vi "S2C_FPGA_WritePort.vi"(8 "Data":u8, 10 "Port":T1(ring), 11 "Connector":enum8{"Conn_0", "Conn_1", "Conn_2"}(ring)) -> ()   [LabVIEW 2015]
uses:
  <vilib>/eio/EIONode/EIONode.xnode
  <vilib>/rvi/eio/common/nirviEmuTemplateMethod_errors.vi
  S2C_FPGA_Global.vi
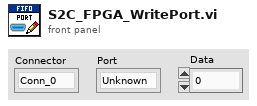
[diagram p1: front panel]
types:
  T1 = enum8{"Unknown", "Port_0", "Port_1", "Port_2", "Port_3", "Port_4"}
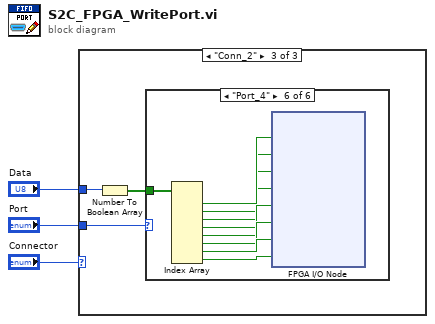
[diagram p0: block diagram]
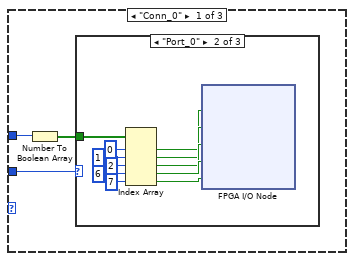
[diagram p2: hidden frame]
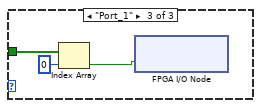
[diagram p4: hidden frame]
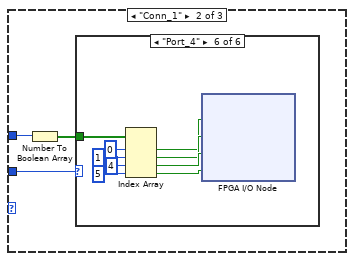
[diagram p5: hidden frame]
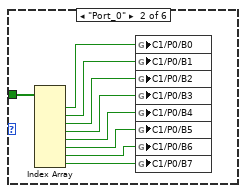
[diagram p7: hidden frame]
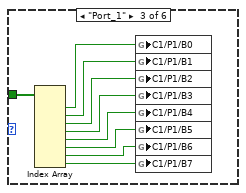
[diagram p8: hidden frame]
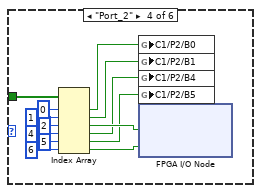
[diagram p9: hidden frame]
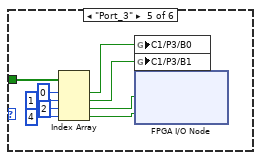
[diagram p10: hidden frame]
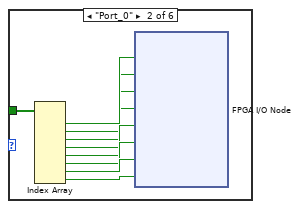
[diagram p12: hidden frame]
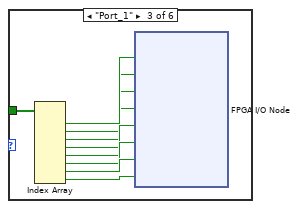
[diagram p13: hidden frame]
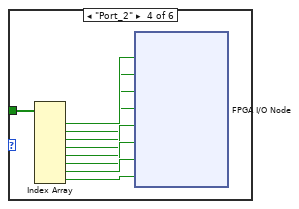
[diagram p14: hidden frame]
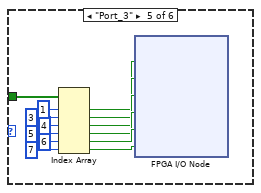
[diagram p15: hidden frame]
diagram:
  n1 = case shown="\"Conn_2\"" "Connector" {
    tunnel: "Data" -> [w6 w23 w75]
    tunnel: "Port" -> [w4 w21 w73]
    frame "Conn_0" {
      n2 = Number To Boolean Array(number=w6) -> (Boolean array=w5:bool[])
      n3 = case shown="\"Port_0\"" w4 {
        tunnel: w5 -> [_ w17 w20]
        frame "Unknown", Default {
        }
        frame "Port_0" {
          n4 = Index Array(array=w17, index #1=0 ("index"), index #2=1 ("index"), index #3=2 ("index"), index #4=6 ("index"), index #5=7 ("index")) -> (element #1=w7:bool, element #2=w8:bool, element #3=w9:bool, element #4=w10:bool, element #5=w11:bool)
          n5 = xnode "FPGA I/O Node"("C0/P0/B0"=w7, "C0/P0/B1"=w8, "C0/P0/B2"=w9, "C0/P0/B6"=w10, "C0/P0/B7"=w11) -> ()  [unwired: 5 in, 5 out]
        }
        frame "Port_1" {
          n6 = Index Array(array=w20, index=0) -> (element=w18:bool)
          n7 = xnode "FPGA I/O Node"("C0/P1/B0"=w18) -> ()  [unwired: 1 in, 1 out]
        }
      }
    }
    frame "Conn_1" {
      n8 = Number To Boolean Array(number=w23) -> (Boolean array=w22:bool[])
      n9 = case shown="\"Port_4\"" w21 {
        tunnel: w22 -> [_ w32 w41 w49 w59 w68]
        frame "Unknown", Default {
        }
        frame "Port_0" {
          n10 = Index Array(array=w32) -> (element #1=w30:bool, element #2=w29:bool, element #3=w28:bool, element #4=w27:bool, element #5=w26:bool, element #6=w25:bool, element #7=w24:bool, element #8=w31:bool)  [unwired: 8 in]
          n11 = global write "S2C_FPGA_Global.vi" "C1/P0/B0"(w30) -> ()
          n12 = global write "S2C_FPGA_Global.vi" "C1/P0/B1"(w29) -> ()
          n13 = global write "S2C_FPGA_Global.vi" "C1/P0/B2"(w28) -> ()
          n14 = global write "S2C_FPGA_Global.vi" "C1/P0/B3"(w27) -> ()
          n15 = global write "S2C_FPGA_Global.vi" "C1/P0/B4"(w26) -> ()
          n16 = global write "S2C_FPGA_Global.vi" "C1/P0/B5"(w25) -> ()
          n17 = global write "S2C_FPGA_Global.vi" "C1/P0/B6"(w24) -> ()
          n18 = global write "S2C_FPGA_Global.vi" "C1/P0/B7"(w31) -> ()
        }
        frame "Port_1" {
          n19 = Index Array(array=w41) -> (element #1=w39:bool, element #2=w38:bool, element #3=w37:bool, element #4=w36:bool, element #5=w35:bool, element #6=w34:bool, element #7=w33:bool, element #8=w40:bool)  [unwired: 8 in]
          n20 = global write "S2C_FPGA_Global.vi" "C1/P1/B0"(w39) -> ()
          n21 = global write "S2C_FPGA_Global.vi" "C1/P1/B1"(w38) -> ()
          n22 = global write "S2C_FPGA_Global.vi" "C1/P1/B2"(w37) -> ()
          n23 = global write "S2C_FPGA_Global.vi" "C1/P1/B3"(w36) -> ()
          n24 = global write "S2C_FPGA_Global.vi" "C1/P1/B4"(w35) -> ()
          n25 = global write "S2C_FPGA_Global.vi" "C1/P1/B5"(w34) -> ()
          n26 = global write "S2C_FPGA_Global.vi" "C1/P1/B6"(w33) -> ()
          n27 = global write "S2C_FPGA_Global.vi" "C1/P1/B7"(w40) -> ()
        }
        frame "Port_2" {
          n28 = Index Array(array=w49, index #1=0 ("index"), index #2=1 ("index"), index #3=2 ("index"), index #4=4 ("index"), index #5=5 ("index"), index #6=6 ("index")) -> (element #1=w48:bool, element #2=w47:bool, element #3=w46:bool, element #4=w44:bool, element #5=w43:bool, element #6=w42:bool)
          n29 = global write "S2C_FPGA_Global.vi" "C1/P2/B0"(w48) -> ()
          n30 = global write "S2C_FPGA_Global.vi" "C1/P2/B1"(w47) -> ()
          n31 = global write "S2C_FPGA_Global.vi" "C1/P2/B4"(w44) -> ()
          n32 = global write "S2C_FPGA_Global.vi" "C1/P2/B5"(w43) -> ()
          n33 = xnode "FPGA I/O Node"("C1/P2/B2"=w46, "C1/P2/B6"=w42) -> ()  [unwired: 2 in, 2 out]
        }
        frame "Port_3" {
          n34 = Index Array(array=w59, index #1=0 ("index"), index #2=1 ("index"), index #3=2 ("index"), index #4=4 ("index")) -> (element #1=w58:bool, element #2=w57:bool, element #3=w56:bool, element #4=w55:bool)
          n35 = global write "S2C_FPGA_Global.vi" "C1/P3/B0"(w58) -> ()
          n36 = global write "S2C_FPGA_Global.vi" "C1/P3/B1"(w57) -> ()
          n37 = xnode "FPGA I/O Node"("C1/P3/B2"=w56, "C1/P3/B4"=w55) -> ()  [unwired: 2 in, 2 out]
        }
        frame "Port_4" {
          n38 = Index Array(array=w68, index #1=0 ("index"), index #2=1 ("index"), index #3=4 ("index"), index #4=5 ("index")) -> (element #1=w64:bool, element #2=w65:bool, element #3=w66:bool, element #4=w67:bool)
          n39 = xnode "FPGA I/O Node"("C1/P4/B0"=w64, "C1/P4/B1"=w65, "C1/P4/B4"=w66, "C1/P4/B5"=w67) -> ()  [unwired: 4 in, 4 out]
        }
      }
    }
    frame "Conn_2" {
      n40 = Number To Boolean Array(number=w75) -> (Boolean array=w74:bool[])
      n41 = case shown="\"Port_4\"" w73 {
        tunnel: w74 -> [_ w84 w93 w102 w110 w124]
        frame "Unknown", Default {
        }
        frame "Port_0" {
          n42 = Index Array(array=w84) -> (element #1=w83:bool, element #2=w76:bool, element #3=w77:bool, element #4=w78:bool, element #5=w79:bool, element #6=w80:bool, element #7=w81:bool, element #8=w82:bool)  [unwired: 8 in]
          n43 = xnode "FPGA I/O Node"("C2/P0/B0"=w83, "C2/P0/B1"=w76, "C2/P0/B2"=w77, "C2/P0/B3"=w78, "C2/P0/B4"=w79, "C2/P0/B5"=w80, "C2/P0/B6"=w81, "C2/P0/B7"=w82) -> ()  [unwired: 8 in, 8 out]
        }
        frame "Port_1" {
          n44 = Index Array(array=w93) -> (element #1=w92:bool, element #2=w85:bool, element #3=w86:bool, element #4=w87:bool, element #5=w88:bool, element #6=w89:bool, element #7=w90:bool, element #8=w91:bool)  [unwired: 8 in]
          n45 = xnode "FPGA I/O Node"("C2/P1/B0"=w92, "C2/P1/B1"=w85, "C2/P1/B2"=w86, "C2/P1/B3"=w87, "C2/P1/B4"=w88, "C2/P1/B5"=w89, "C2/P1/B6"=w90, "C2/P1/B7"=w91) -> ()  [unwired: 8 in, 8 out]
        }
        frame "Port_2" {
          n46 = Index Array(array=w102) -> (element #1=w101:bool, element #2=w94:bool, element #3=w95:bool, element #4=w96:bool, element #5=w97:bool, element #6=w98:bool, element #7=w99:bool, element #8=w100:bool)  [unwired: 8 in]
          n47 = xnode "FPGA I/O Node"("C2/P2/B0"=w101, "C2/P2/B1"=w94, "C2/P2/B2"=w95, "C2/P2/B3"=w96, "C2/P2/B4"=w97, "C2/P2/B5"=w98, "C2/P2/B6"=w99, "C2/P2/B7"=w100) -> ()  [unwired: 8 in, 8 out]
        }
        frame "Port_3" {
          n48 = Index Array(array=w110, index #1=1 ("index"), index #2=3 ("index"), index #3=4 ("index"), index #4=5 ("index"), index #5=6 ("index"), index #6=7 ("index")) -> (element #1=w103:bool, element #2=w104:bool, element #3=w105:bool, element #4=w106:bool, element #5=w107:bool, element #6=w108:bool)
          n49 = xnode "FPGA I/O Node"("C2/P3/B1"=w103, "C2/P3/B3"=w104, "C2/P3/B4"=w105, "C2/P3/B5"=w106, "C2/P3/B6"=w107, "C2/P3/B7"=w108) -> ()  [unwired: 6 in, 6 out]
        }
        frame "Port_4" {
          n50 = Index Array(array=w124) -> (element #1=w123:bool, element #2=w116:bool, element #3=w117:bool, element #4=w118:bool, element #5=w119:bool, element #6=w120:bool, element #7=w121:bool, element #8=w122:bool)  [unwired: 8 in]
          n51 = xnode "FPGA I/O Node"("C2/P4/B0"=w123, "C2/P4/B1"=w116, "C2/P4/B2"=w117, "C2/P4/B3"=w118, "C2/P4/B4"=w119, "C2/P4/B5"=w120, "C2/P4/B6"=w121, "C2/P4/B7"=w122) -> ()  [unwired: 8 in, 8 out]
        }
      }
    }
  }
